vi "Parse CSV to Doubles Array LabVIEW 2012 NI Verified.vi"(11 "file path (use dialog)":path) -> (1 "Numeric Array":dbl[][](array[numeric]), 2 "Header":string, 3 "text":string)   [LabVIEW 2020]
doc: "This example VI reads a CSV file with header and gets the data in a double array"
panel:
  in  "End Of Header":string="--"
  # "Overview: This example VI reads a CSV file with header and gets the data in a double array \nRequirements: LabVIEW 2012 (or compatible)\nInstructions:\n1. Select the CSV file\n2. Write the end of the header. (The \"End Of Header\" input must be the same string used in the csv file  as End Of Header) \n3. Run the VI"
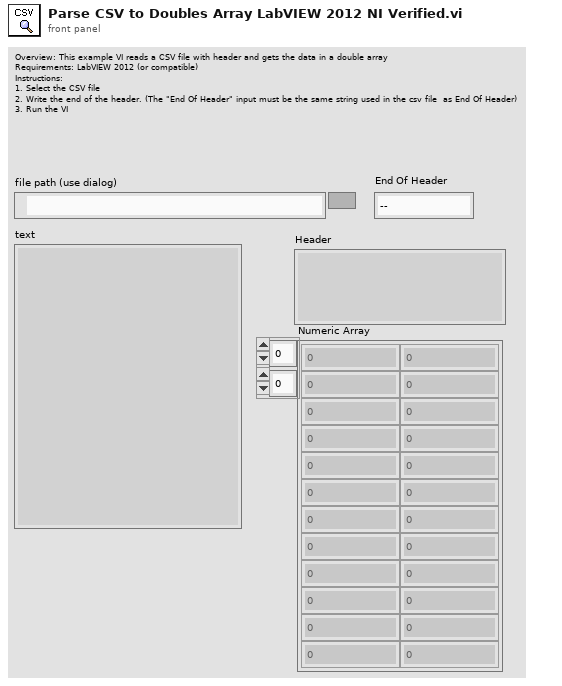
[diagram p1: front panel]
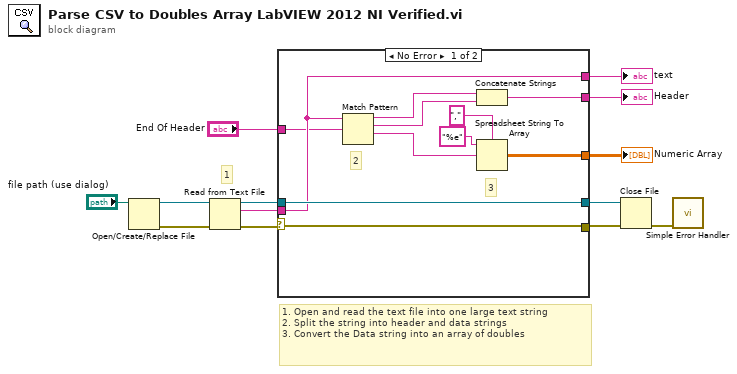
[diagram p0: block diagram]
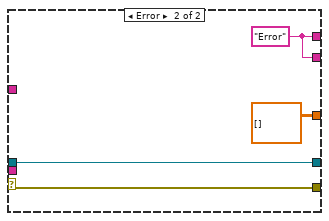
[diagram p2: hidden frame]
diagram:
  # "1"
  # "1. Open and read the text file into one large text string\n2. Split the string into header and data strings\n3. Convert the Data string into an array of doubles"
  n1 = Open/Create/Replace File(file path (use dialog)="file path (use dialog)") -> (refnum out=w12:refnum<file>, error out=w11:errorcluster)  [unwired: 5 in, 1 out]
  n2 = Read from Text File(file (use dialog)=w12, error in=w11) -> (refnum out=w7:refnum<file>, text=w10:string, error out=w9:errorcluster)  [unwired: 2 in, 1 out]
  n3 = case shown="No Error" w9 {
    selector: w9 -> [w19 w28]
    tunnel: w10 -> [w17 _]
    tunnel: [w19 w28] -> w8
    tunnel: w7 -> [w18 w27]
    tunnel: [w18 w27] -> w6
    tunnel: [w17 w26] -> w4
    tunnel: [w16 w26] -> w3
    tunnel: [w15 dbl[][] []] -> w2
    tunnel: "End Of Header" -> [w14 _]
    frame No Error {
      # "3"
      # "2"
      n4 = Match Pattern(string=w17, regular expression=w14) -> (before substring=w21:string, match substring=w20:string, after substring=w24:string)  [unwired: 1 in, 1 out]
      n5 = Concatenate Strings(w21, w20) -> (w16:string)
      n6 = Spreadsheet String To Array(delimiter (Tab)=",", format string="%e", spreadsheet string=w24) -> (array=w15:dbl[][])  [unwired: 1 in]
    }
    frame Error {
      w26 = "Error"
    }
  }
  "text" <- w4
  "Header" <- w3
  "Numeric Array" <- w2
  n7 = Close File(refnum=w6, error in=w8) -> (error out=w5:errorcluster)  [unwired: 1 out]
  n8 = call <vilib>:"Simple Error Handler.vi"("error in (no error)"=w5) -> ()  [unwired: 4 in, 5 out]
